vi "VCI_BOARD_INFO1_CONVERT.vi"(1 "VCI_BOARD_INFO1":T2) -> (0 "VCI_BOARD_INFO1_1":T1)   [LabVIEW 2018, in "ControlCan.lvlib"]
uses:
  ControlCan.lvlib
  VCI_BOARD_INFO1.ctl
  VCI_BOARD_INFO1_1.ctl
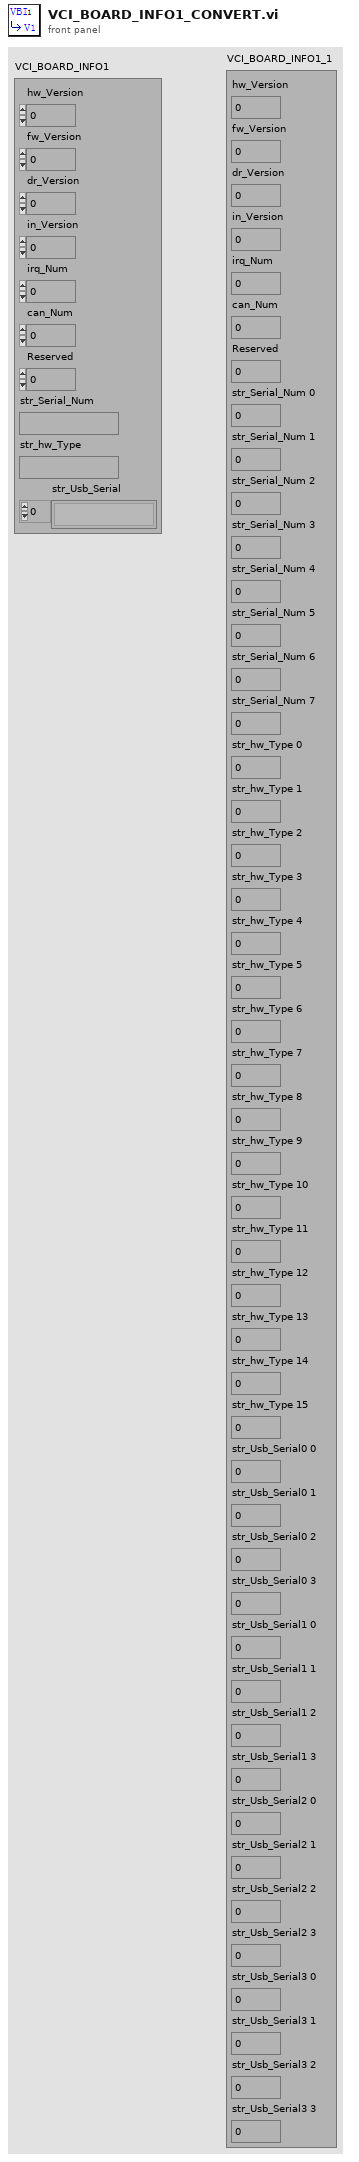
[diagram p1: front panel]
types:
  T1 = typedef "ControlCAN.lvlib/VCI_BOARD_INFO1_1.ctl" = cluster{"hw_Version":u16, "fw_Version":u16, "dr_Version":u16, "in_Version":u16, "irq_Num":u16, "can_Num":u8, "Reserved":u8, "str_Serial_Num 0":u8, "str_Serial_Num 1":u8, "str_Serial_Num 2":u8, "str_Serial_Num 3":u8, "str_Serial_Num 4":u8, "str_Serial_Num 5":u8, "str_Serial_Num 6":u8, "str_Serial_Num 7":u8, "str_hw_Type 0":u8, "str_hw_Type 1":u8, "str_hw_Type 2":u8, "str_hw_Type 3":u8, "str_hw_Type 4":u8, "str_hw_Type 5":u8, "str_hw_Type 6":u8, "str_hw_Type 7":u8, "str_hw_Type 8":u8, "str_hw_Type 9":u8, "str_hw_Type 10":u8, "str_hw_Type 11":u8, "str_hw_Type 12":u8, "str_hw_Type 13":u8, "str_hw_Type 14":u8, "str_hw_Type 15":u8, "str_Usb_Serial0 0":u8, "str_Usb_Serial0 1":u8, "str_Usb_Serial0 2":u8, "str_Usb_Serial0 3":u8, "str_Usb_Serial1 0":u8, "str_Usb_Serial1 1":u8, "str_Usb_Serial1 2":u8, "str_Usb_Serial1 3":u8, "str_Usb_Serial2 0":u8, "str_Usb_Serial2 1":u8, "str_Usb_Serial2 2":u8, "str_Usb_Serial2 3":u8, "str_Usb_Serial3 0":u8, "str_Usb_Serial3 1":u8, "str_Usb_Serial3 2":u8, "str_Usb_Serial3 3":u8}
  T2 = typedef "ControlCAN.lvlib/VCI_BOARD_INFO1.ctl" = cluster{"hw_Version":u16, "fw_Version":u16, "dr_Version":u16, "in_Version":u16, "irq_Num":u16, "can_Num":u8, "Reserved":u8, "str_Serial_Num":string, "str_hw_Type":string, "str_Usb_Serial":string[]}
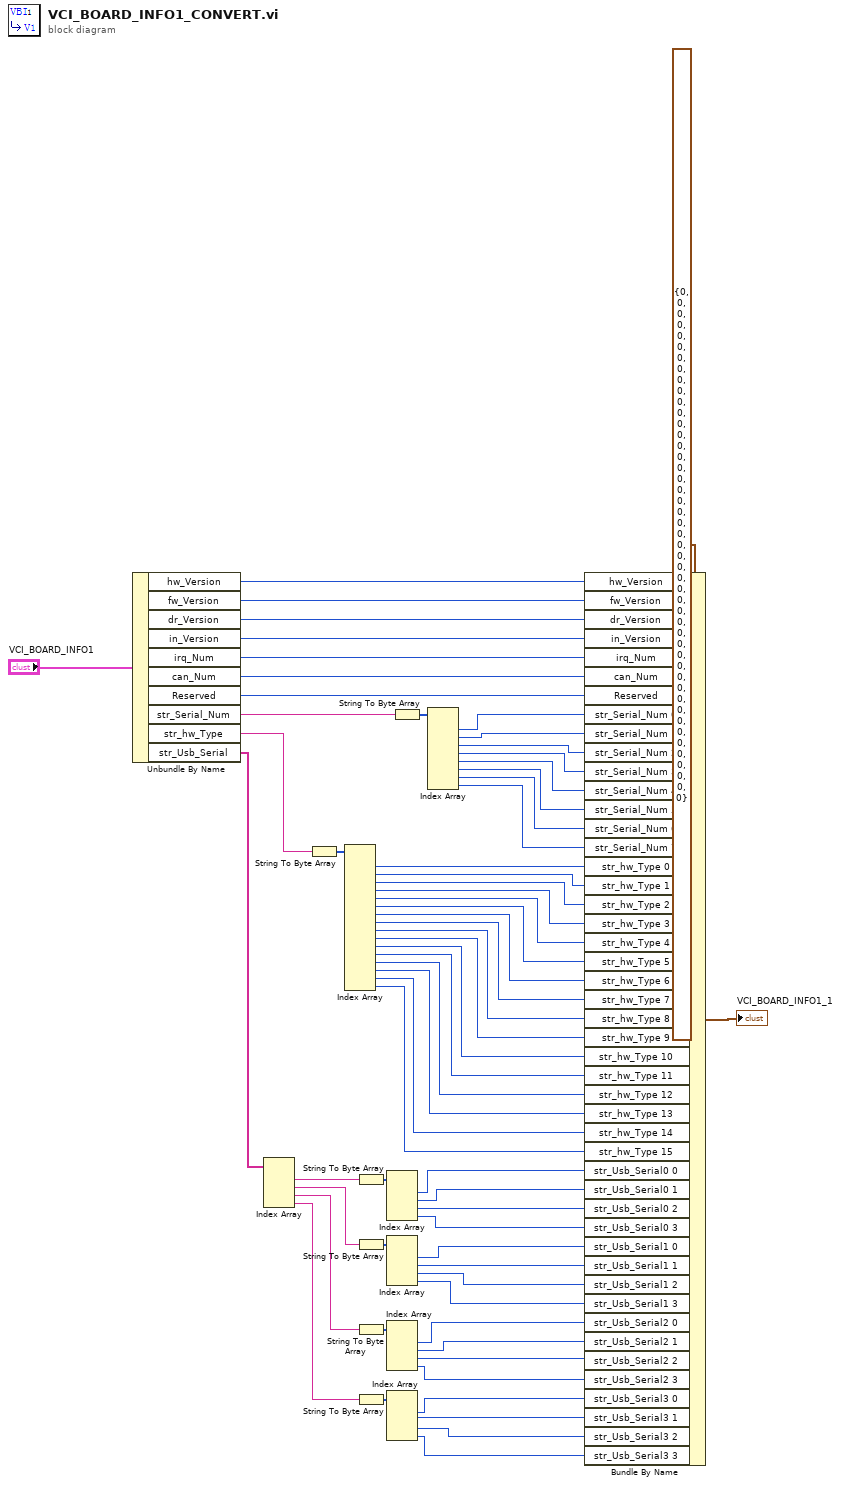
[diagram p0: block diagram]
diagram:
  n1 = Unbundle By Name("VCI_BOARD_INFO1") -> ("hw_Version"=w61:u16, "fw_Version"=w60:u16, "dr_Version"=w59:u16, "in_Version"=w58:u16, "irq_Num"=w57:u16, "can_Num"=w56:u8, "Reserved"=w55:u8, "str_Serial_Num"=w54:string, "str_hw_Type"=w43:string, "str_Usb_Serial"=w26:string[])
  n2 = Index Array(array=w26) -> (element #1=w25:string, element #2=w18:string, element #3=w12:string, element #4=w6:string)  [unwired: 4 in]
  n3 = String To Byte Array(string=w43) -> (unsigned byte array=w44:u8[])
  n4 = Index Array(array=w44) -> (element #1=w42:u8, element #2=w41:u8, element #3=w40:u8, element #4=w39:u8, element #5=w38:u8, element #6=w37:u8, element #7=w36:u8, element #8=w35:u8, element #9=w34:u8, element #10=w33:u8, element #11=w32:u8, element #12=w31:u8, element #13=w30:u8, element #14=w29:u8, element #15=w28:u8, element #16=w27:u8)  [unwired: 16 in]
  n5 = String To Byte Array(string=w25) -> (unsigned byte array=w24:u8[])
  n6 = String To Byte Array(string=w18) -> (unsigned byte array=w19:u8[])
  n7 = String To Byte Array(string=w12) -> (unsigned byte array=w13:u8[])
  n8 = String To Byte Array(string=w6) -> (unsigned byte array=w7:u8[])
  n9 = Index Array(array=w24) -> (element #1=w23:u8, element #2=w22:u8, element #3=w21:u8, element #4=w20:u8)  [unwired: 4 in]
  n10 = Index Array(array=w19) -> (element #1=w17:u8, element #2=w16:u8, element #3=w15:u8, element #4=w14:u8)  [unwired: 4 in]
  n11 = Index Array(array=w13) -> (element #1=w11:u8, element #2=w10:u8, element #3=w9:u8, element #4=w8:u8)  [unwired: 4 in]
  n12 = Index Array(array=w7) -> (element #1=w5:u8, element #2=w4:u8, element #3=w3:u8, element #4=w2:u8)  [unwired: 4 in]
  n13 = String To Byte Array(string=w54) -> (unsigned byte array=w53:u8[])
  n14 = Index Array(array=w53) -> (element #1=w52:u8, element #2=w51:u8, element #3=w50:u8, element #4=w49:u8, element #5=w48:u8, element #6=w47:u8, element #7=w46:u8, element #8=w45:u8)  [unwired: 8 in]
  n15 = Bundle By Name(cluster=T1 {"hw_Version"=0, "fw_Version"=0, "dr_Version"=0, "in_Version"=0, "irq_Num"=0, "can_Num"=0, "Reserved"=0, "str_Serial_Num 0"=0, "str_Serial_Num 1"=0, "str_Serial_Num 2"=0, "str_Serial_Num 3"=0, "str_Serial_Num 4"=0, "str_Serial_Num 5"=0, "str_Serial_Num 6"=0, "str_Serial_Num 7"=0, "str_hw_Type 0"=0, "str_hw_Type 1"=0, "str_hw_Type 2"=0, "str_hw_Type 3"=0, "str_hw_Type 4"=0, "str_hw_Type 5"=0, "str_hw_Type 6"=0, "str_hw_Type 7"=0, "str_hw_Type 8"=0, "str_hw_Type 9"=0, "str_hw_Type 10"=0, "str_hw_Type 11"=0, "str_hw_Type 12"=0, "str_hw_Type 13"=0, "str_hw_Type 14"=0, "str_hw_Type 15"=0, "str_Usb_Serial0 0"=0, "str_Usb_Serial0 1"=0, "str_Usb_Serial0 2"=0, "str_Usb_Serial0 3"=0, "str_Usb_Serial1 0"=0, "str_Usb_Serial1 1"=0, "str_Usb_Serial1 2"=0, "str_Usb_Serial1 3"=0, "str_Usb_Serial2 0"=0, "str_Usb_Serial2 1"=0, "str_Usb_Serial2 2"=0, "str_Usb_Serial2 3"=0, "str_Usb_Serial3 0"=0, "str_Usb_Serial3 1"=0, "str_Usb_Serial3 2"=0, "str_Usb_Serial3 3"=0} ("VCI_BOARD_INFO1_1"), "hw_Version"=w61, "fw_Version"=w60, "dr_Version"=w59, "in_Version"=w58, "irq_Num"=w57, "can_Num"=w56, "Reserved"=w55, "str_Serial_Num 0"=w52, "str_Serial_Num 1"=w51, "str_Serial_Num 2"=w50, "str_Serial_Num 3"=w49, "str_Serial_Num 4"=w48, "str_Serial_Num 5"=w47, "str_Serial_Num 6"=w46, "str_Serial_Num 7"=w45, "str_hw_Type 0"=w42, "str_hw_Type 1"=w41, "str_hw_Type 2"=w40, "str_hw_Type 3"=w39, "str_hw_Type 4"=w38, "str_hw_Type 5"=w37, "str_hw_Type 6"=w36, "str_hw_Type 7"=w35, "str_hw_Type 8"=w34, "str_hw_Type 9"=w33, "str_hw_Type 10"=w32, "str_hw_Type 11"=w31, "str_hw_Type 12"=w30, "str_hw_Type 13"=w29, "str_hw_Type 14"=w28, "str_hw_Type 15"=w27, "str_Usb_Serial0 0"=w23, "str_Usb_Serial0 1"=w22, "str_Usb_Serial0 2"=w21, "str_Usb_Serial0 3"=w20, "str_Usb_Serial1 0"=w17, "str_Usb_Serial1 1"=w16, "str_Usb_Serial1 2"=w15, "str_Usb_Serial1 3"=w14, "str_Usb_Serial2 0"=w11, "str_Usb_Serial2 1"=w10, "str_Usb_Serial2 2"=w9, "str_Usb_Serial2 3"=w8, "str_Usb_Serial3 0"=w5, "str_Usb_Serial3 1"=w4, "str_Usb_Serial3 2"=w3, "str_Usb_Serial3 3"=w2) -> (→"VCI_BOARD_INFO1_1":T1)
